vi "Database.File.Read.vi"(1 "Values":T1 {"Products"."Values" format="%.3f"}, 8 "error in (no error)":errorcluster, 9 "B?":bool, 10 "FileName":string, 11 "Data in":T4={"Status"={"Run"=FALSE, "Handle"=0, "ConnTS"=timestamp(0 s since 1904-01-01), "DbTime"=timestamp(0 s since 1904-01-01), "DbTimeCode"=0.0}, "Sets"={"Enable"=FALSE, "R/W"=FALSE, "LogDebug"=FALSE, "ConnString"="", "ProductionLine"="", "SystemName1"="T075", "SystemName2"=""}, "Results"={"Status"=enum."-", "Service"=FALSE, "Ref"="", "Serial"="", "ID"={"processId"=0, "systemId"=0, "processStepId"=0, "wabcoPartId"=0}, "P"={"c_id"="", "productId"="", "processId"=0, "statusId"=0, "startTime"="", "endTime"=""}, "PS"={"c_id"="", "processResultId"="", "processStepId"=0, "statusId"=0, "operatorId"=0, "startTime"="", "endTime"=""}, "TS"=[]}, "Variant"={"Found"=FALSE, "Ref"="", "ID"={"processId"=0, "systemId"=0, "processStepId"=0, "wabcoPartId"=0}, "PP"=[], "TS"=[]}} {"Variant"."TS"."TV"."minimum" format="%#.3f"; "Variant"."TS"."TV"."maximum" format="%#.3f"; "Variant"."TS"."TP"."value" format="%#.3f"}) -> (0 "error out":errorcluster, 3 "Data out":T4={"Status"={"Run"=FALSE, "Handle"=0, "ConnTS"=timestamp(0 s since 1904-01-01), "DbTime"=timestamp(0 s since 1904-01-01), "DbTimeCode"=0.0}, "Sets"={"Enable"=FALSE, "R/W"=FALSE, "LogDebug"=FALSE, "ConnString"="", "ProductionLine"="", "SystemName1"="T075", "SystemName2"=""}, "Results"={"Status"=enum."-", "Service"=FALSE, "Ref"="", "Serial"="", "ID"={"processId"=0, "systemId"=0, "processStepId"=0, "wabcoPartId"=0}, "P"={"c_id"="", "productId"="", "processId"=0, "statusId"=0, "startTime"="", "endTime"=""}, "PS"={"c_id"="", "processResultId"="", "processStepId"=0, "statusId"=0, "operatorId"=0, "startTime"="", "endTime"=""}, "TS"=[]}, "Variant"={"Found"=FALSE, "Ref"="", "ID"={"processId"=0, "systemId"=0, "processStepId"=0, "wabcoPartId"=0}, "PP"=[], "TS"=[]}} {"Variant"."TS"."TV"."minimum" format="%#.3f"; "Variant"."TS"."TV"."maximum" format="%#.3f"; "Variant"."TS"."TP"."value" format="%#.3f"})   [LabVIEW 2016]
uses:
  Global/ApplicationGlobal.vi
  Database.Main.Data.Status.ctl
  Database.Main.Data.Sets.ctl
  Database.Main.Data.ctl
  Sequence/Sequence.Step.Status.ctl
  ProdaNG/Controls/ProdaNG.ProcessResult.ctl
  ProdaNG/Controls/ProdaNG.ProcessStepResult.ctl
  ProdaNG/Controls/ProdaNG.TestStepResult.ctl
  ProdaNG/Controls/ProdaNG.TestValueResult.ctl
  ProdaNG/Controls/ProdaNG.Identification.ctl
  ProdaNG/Controls/ProdaNG.TestStepParam.ctl
  ProdaNG/Controls/ProdaNG.ProcessStepParam.ctl
  Database.Main.Data.Results.ctl
  ProdaNG/Controls/ProdaNG.TestValue.ctl
  ProdaNG/Controls/ProdaNG.TestStep.ctl
  Database.Main.Data.Variant.ctl
  Database.Main.Results.Product.ctl
  Database.Main.Results.Variant.ctl
panel:
  out "groups":string[](array[string])
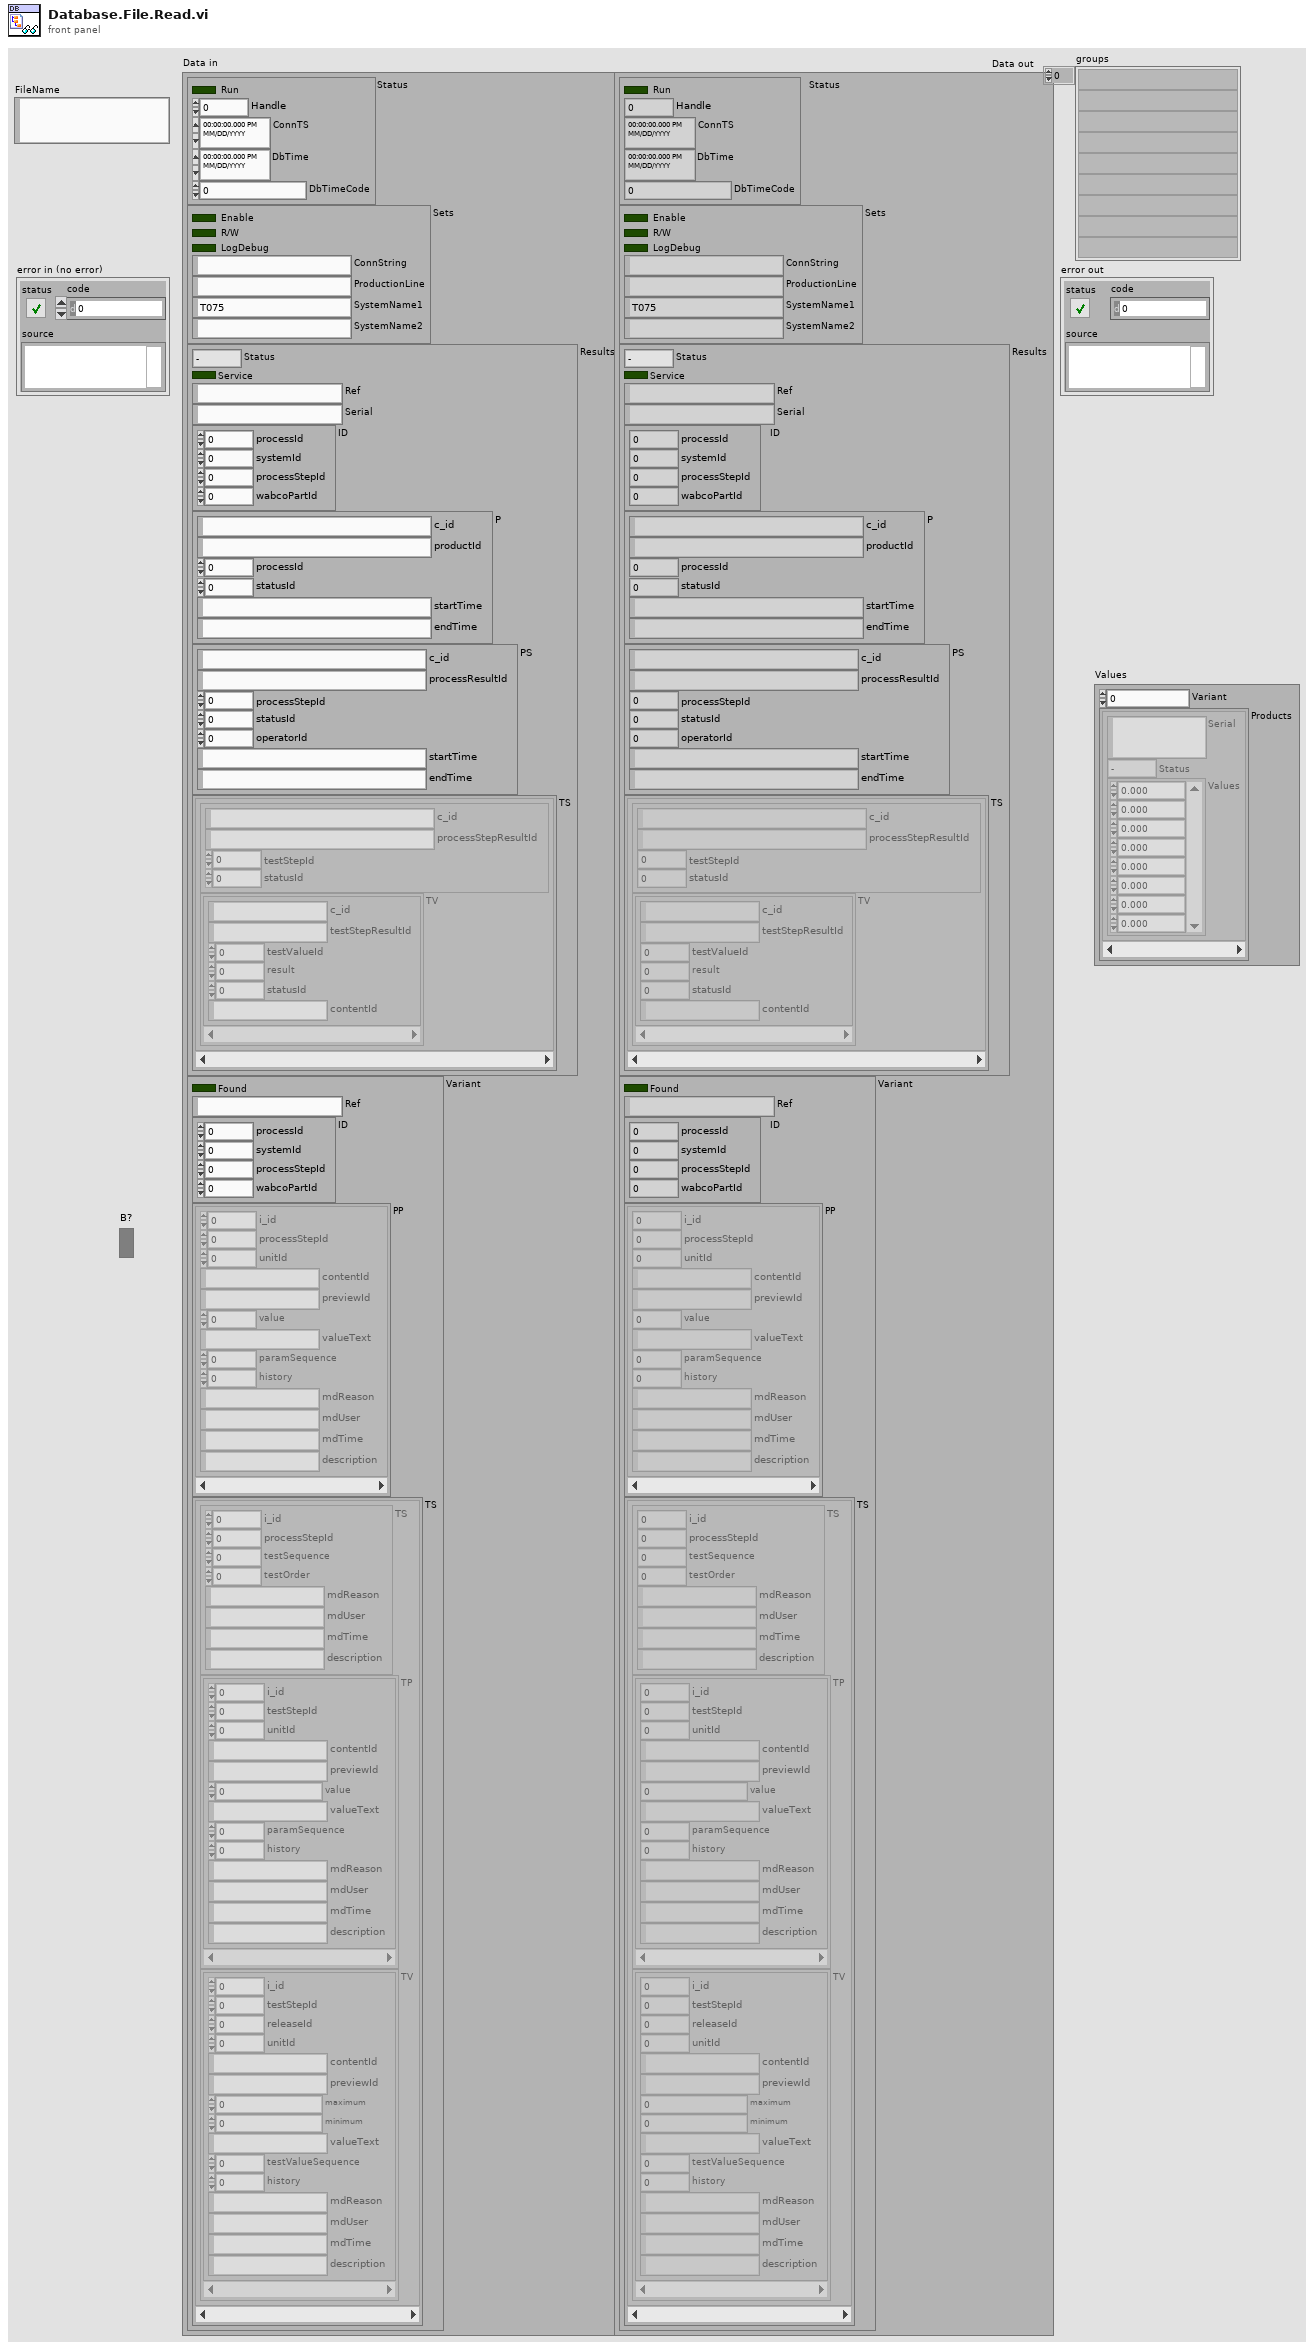
[diagram p1: front panel]
types:
  T1 = typedef "Database.Main.Results.Variant.ctl" = cluster{"Variant":u64, "Products":T2[]}
  T2 = typedef "Database.Main.Results.Product.ctl" = cluster{"Serial":string, "Status":T3, "Values":dbl[]}
  T3 = typedef "Sequence.Step.Status.ctl" = enum16{"-", "Pending", "Running", "Skipped", "Passed", "Failed", "Done", "Error", "Aborted", "Stopped"}
  T4 = typedef "Database.Main.Data.ctl" = cluster{"Status":T5, "Sets":T6, "Results":T7, "Variant":T13}
  T5 = typedef "Database.Main.Data.Status.ctl" = cluster{"Run":bool, "Handle":i32, "ConnTS":timestamp, "DbTime":timestamp, "DbTimeCode":dbl}
  T6 = typedef "Database.Main.Data.Sets.ctl" = cluster{"Enable":bool, "R/W":bool, "LogDebug":bool, "ConnString":string, "ProductionLine":string, "SystemName1":string, "SystemName2":string}
  T7 = typedef "Database.Main.Data.Results.ctl" = cluster{"Status":T3, "Service":bool, "Ref":string, "Serial":string, "ID":T8, "P":T9, "PS":T10, "TS":cluster{"TS":T11, "TV":T12[]}[]}
  T8 = typedef "ProdaNG.Identification.ctl" = cluster{"processId":i32, "systemId":i32, "processStepId":i32, "wabcoPartId":i32}
  T9 = typedef "ProdaNG.ProcessResult.ctl" = cluster{"c_id":string, "productId":string, "processId":i32, "statusId":i32, "startTime":string, "endTime":string}
  T10 = typedef "ProdaNG.ProcessStepResult.ctl" = cluster{"c_id":string, "processResultId":string, "processStepId":i32, "statusId":i32, "operatorId":i32, "startTime":string, "endTime":string}
  T11 = typedef "ProdaNG.TestStepResult.ctl" = cluster{"c_id":string, "processStepResultId":string, "testStepId":i32, "statusId":i32}
  T12 = typedef "ProdaNG.TestValueResult.ctl" = cluster{"c_id":string, "testStepResultId":string, "testValueId":i32, "result":dbl, "statusId":i32, "contentId":string}
  T13 = typedef "Database.Main.Data.Variant.ctl" = cluster{"Found":bool, "Ref":string, "ID":T8, "PP":T14[], "TS":cluster{"TS":T15, "TP":T16[], "TV":T17[]}[]}
  T14 = typedef "ProdaNG.ProcessStepParam.ctl" = cluster{"i_id":i32, "processStepId":i32, "unitId":i32, "contentId":string, "previewId":string, "value":dbl, "valueText":string, "paramSequence":i32, "history":i32, "mdReason":string, "mdUser":string, "mdTime":string, "description":string}
  T15 = typedef "ProdaNG.TestStep.ctl" = cluster{"i_id":i32, "processStepId":i32, "testSequence":i32, "testOrder":i32, "mdReason":string, "mdUser":string, "mdTime":string, "description":string}
  T16 = typedef "ProdaNG.TestStepParam.ctl" = cluster{"i_id":i32, "testStepId":i32, "unitId":i32, "contentId":string, "previewId":string, "value":dbl, "valueText":string, "paramSequence":i32, "history":i32, "mdReason":string, "mdUser":string, "mdTime":string, "description":string}
  T17 = typedef "ProdaNG.TestValue.ctl" = cluster{"i_id":i32, "testStepId":i32, "releaseId":i32, "unitId":i32, "contentId":string, "previewId":string, "maximum":dbl, "minimum":dbl, "valueText":string, "testValueSequence":i32, "history":i32, "mdReason":string, "mdUser":string, "mdTime":string, "description":string}
  T18 = enum16{"open", "open or create", "create or replace", "create", "open (read-only)"}
  T19 = cluster{"LogName":string, "Name":string, "Status":T3, "Step":T11, "Values":cluster{"Name":string, "Status":T3, "Result":T12}[]}[]
  T20 = typedef "Sequence.SeqMode.ctl" = enum16{"Auto", "Step", "CG"}
  T21 = cluster{"Name":string, "Status":T3, "Result":T12}[]
  T22 = cluster{"Name":string, "Status":T3, "Result":T12}
  T23 = cluster{"LogName":string, "Name":string, "Status":T3, "Step":T11, "Values":cluster{"Name":string, "Status":T3, "Result":T12}[]}
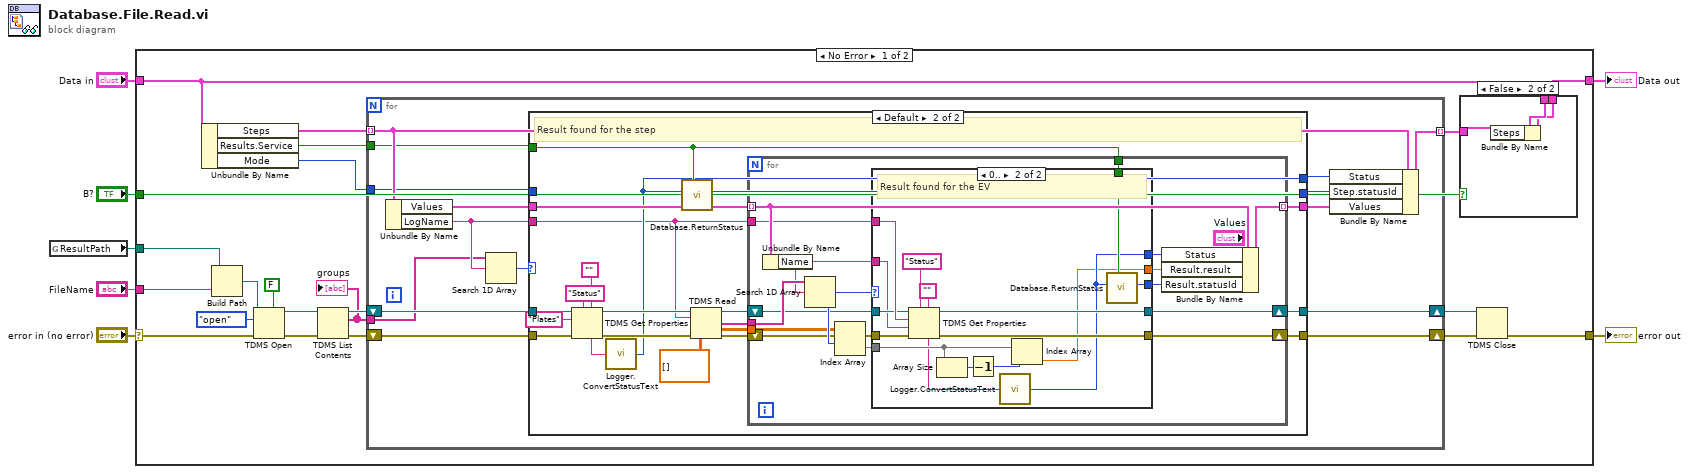
[diagram p0: block diagram]
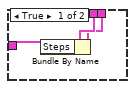
[diagram p2: hidden frame]
diagram:
  n1 = global read "ApplicationGlobal.vi" "ResultPath"() -> (w4:path)
  n2 = case shown="No Error" "error in (no error)" {
    selector: "error in (no error)" -> [w26 w109]
    tunnel: [w19 w109] -> w7
    tunnel: "FileName" -> [w24 _]
    tunnel: w4 -> [w23 _]
    tunnel: "Data in" -> [w18 w108]
    tunnel: [w17 w108] -> w2
    tunnel: "B?" -> [w8 _]
    frame No Error {
      n3 = Unbundle By Name(w18) -> ("Steps"=w16:T19, "Results.Service"=w11:bool, "Mode"=w12:T20)
      n4 = Build Path(base path=w23, name or relative path=w24) -> (appended path=w22:path)
      n5 = TDMS Open(5:FALSE ("create index file? (T)"), 8:w26, 10:T18."open" ("operation (0:open)"), 11:w22) -> (0:w13:errorcluster, 3:w14:refnum<k34>)  [unwired: 3 in]
      n6 = TDMS List Contents(4:w13, 7:w14) -> (0:w9:errorcluster, 2:w10:string[], 3:w25:refnum<k34>)  [unwired: 1 in, 1 out]
      "groups" <- w10
      n7 = for {
        shift-right: [w44] -> w21
        shift-left: w9 -> [w49]
        shift-right: [w45] -> w20
        shift-left: w25 -> [w38]
        tunnel: w10 -> [w35]
        tunnel: w16 -> [w48] mode=indexing
        tunnel: [w47] -> w15 mode=indexing
        tunnel: w12 -> [w41]
        tunnel: w11 -> [w40]
        n8 = Unbundle By Name(w48) -> ("Values"=w39:T21, "LogName"=w37:string)
        n9 = Search 1D Array(1D array=w35, element=w37) -> (index of element=w36:i32)  [unwired: 1 in]
        n10 = case shown="Default" w36 {
          tunnel: w38 -> [w52 w67]
          tunnel: w49 -> [w51 w68]
          tunnel: [_ w55] -> w46
          tunnel: w39 -> [w50 w73]
          tunnel: [w52 w59] -> w45
          tunnel: [w51 w58] -> w44
          tunnel: [w50 w69] -> w43
          tunnel: w41 -> [_ _]
          tunnel: [_ w64] -> w42
          tunnel: w40 -> [_ w63]
          tunnel: w37 -> [_ w54]
          frame -1 {
            # "No results found for the step (skipped)"
          }
          frame Default {
            # "Result found for the step"
            n11 = TDMS Get Properties(5:"", 7:"Status" ("property name"), 8:w68, 10:"Plates" ("group name"), 11:w67) -> (0:w65:errorcluster, 3:w66:refnum<k34>, 4:w56:string)  [unwired: 1 in, 3 out]
            n12 = call "Logger.ConvertStatusText.vi"("Status string"=w56) -> ("Status"=w55:T3)
            n13 = call "Database.ReturnStatus.vi"("service"=w63, "Status"=w55) -> ("Step.statusId"=w64:i32)  [unwired: 8 in, 1 out]
            n14 = TDMS Read(0:w66, 5:w54, 11:w65, 12:dbl[][] []) -> (4:w57:refnum<k34>, 8:w71:string[], 10:w70:dbl[][], 15:w60:errorcluster)  [unwired: 4 in, 2 out]
            n15 = for {
              tunnel: w73 -> [w89] mode=indexing
              tunnel: w71 -> [w82]
              tunnel: w70 -> [w87]
              tunnel: [w84] -> w69 mode=indexing
              tunnel: w63 -> [w81]
              shift-right: [w76] -> w59
              shift-left: w57 -> [w78]
              shift-right: [w77] -> w58
              shift-left: w60 -> [w79]
              tunnel: w54 -> [w75]
              n16 = Unbundle By Name(w89) -> ("Name"=w74:string)
              n17 = Search 1D Array(1D array=w82, element=w74) -> (index of element=w88:i32)  [unwired: 1 in]
              n18 = Index Array(array=w87, index (row)=w88) -> (element=w80:dbl[])  [unwired: 1 in]
              n19 = case shown="0.." w88 {
                tunnel: w80 -> [_ w105]
                tunnel: [_ w93] -> w86
                tunnel: [_ w92] -> w85
                tunnel: [_ w107] -> w83
                tunnel: w81 -> [_ w106]
                tunnel: w79 -> [w91 w102]
                tunnel: w78 -> [w90 w96]
                tunnel: [w91 w100] -> w77
                tunnel: [w90 w101] -> w76
                tunnel: w75 -> [_ w97]
                tunnel: w74 -> [_ w95]
                frame Default {
                  # "No result found for the EV"
                }
                frame 0.. {
                  # "Result found for the EV"
                  n20 = TDMS Get Properties(5:"", 7:"Status" ("property name"), 8:w102, 9:w95, 10:w97, 11:w96) -> (0:w100:errorcluster, 3:w101:refnum<k34>, 4:w94:string)  [unwired: 3 out]
                  n21 = Array Size(array=w105) -> (size(s)=w104:i32)
                  n22 = Decrement(x=w104) -> (x-1=w103:i32)
                  n23 = call "Logger.ConvertStatusText.vi"("Status string"=w94) -> ("Status"=w93:T3)
                  n24 = Index Array(array=w105, index=w103) -> (element=w92:dbl)
                  n25 = call "Database.ReturnStatus.vi"("service"=w106, "Status"=w93) -> ("Step.statusId"=w107:i32)  [unwired: 8 in, 1 out]
                }
              }
              n26 = Bundle By Name(cluster=w89, "Status"=w86, "Result.result"=w85, "Result.statusId"=w83) -> (w84:T22)
            }
          }
        }
        n27 = Bundle By Name(cluster=w48, "Status"=w46, "Step.statusId"=w42, "Values"=w43) -> (w47:T23)
      }
      n28 = case shown="False" w8 {
        tunnel: w18 -> [w31 w34]
        tunnel: [w30 w33] -> w17
        tunnel: w15 -> [w29 w32]
        frame True {
          n29 = Bundle By Name(cluster=w31, "Steps"=w29) -> (w30:T4)
        }
        frame False {
          n30 = Bundle By Name(cluster=w34, "Steps"=w32) -> (w33:T4)
        }
      }
      n31 = TDMS Close(8:w21, 11:w20) -> (0:w19:errorcluster)  [unwired: 1 out]
    }
    frame Error {
    }
  }
  "error out" <- w7
  "Data out" <- w2
